vi "rad_FTP Get File Wrapper.vi"(4 "active (F)":bool, 5 "password":string, 6 "binary (T)":bool=TRUE, 8 "error in (no error)":errorcluster, 9 "local path":path=path "C:/Users/bsnover/Desktop/lvappimage.info", 10 "remote path":string="c:\\lvappimage.info", 11 "Target settings":T1={"Hostname"="", "Serial number"="", "Product name"="", "Product code"=0, "System status"="", "Credential type"=enum."None/Unlocked", "User added?"=FALSE, "Primary NIC"={"MAC address"="", "IP Address Request Mode"=2, "IP address"="", "Subnet mask"="", "Gateway"="", "DNS server"=""}} {"Primary NIC"."IP Address Request Mode" items=["Static"=1, "DHCP/Link-Local"=2, "Link-Local Only"=4, "DHCP Only"=8]}) -> (0 "error out":errorcluster)   [LabVIEW 2020]
uses:
  <vilib>/nisyscfg/nisyscfg.lvlib
  <vilib>/nisyscfg/Close (System).vi
  <vilib>/FTP/NI_FTP.lvlib
  Targets/TypeDefs/rad_Target Information.ctl
  Targets/TypeDefs/rad_Target Network Settings.ctl
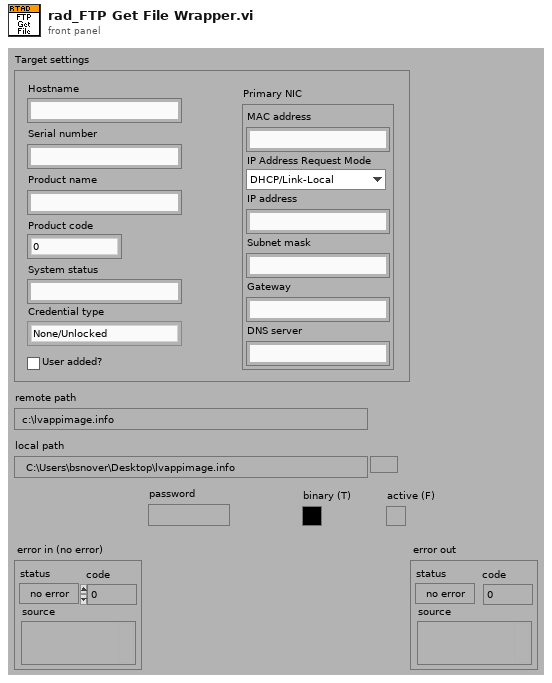
[diagram p1: front panel]
types:
  T1 = typedef "rad_Target Information.ctl" = cluster{"Hostname":string, "Serial number":string, "Product name":string, "Product code":i32, "System status":string, "Credential type":enum16{"None/Unlocked", "FTP Password", "NIAuth Credentials"}, "User added?":bool, "Primary NIC":T2}
  T2 = typedef "rad_Target Network Settings.ctl" = cluster{"MAC address":string, "IP Address Request Mode":i32, "IP address":string, "Subnet mask":string, "Gateway":string, "DNS server":string}
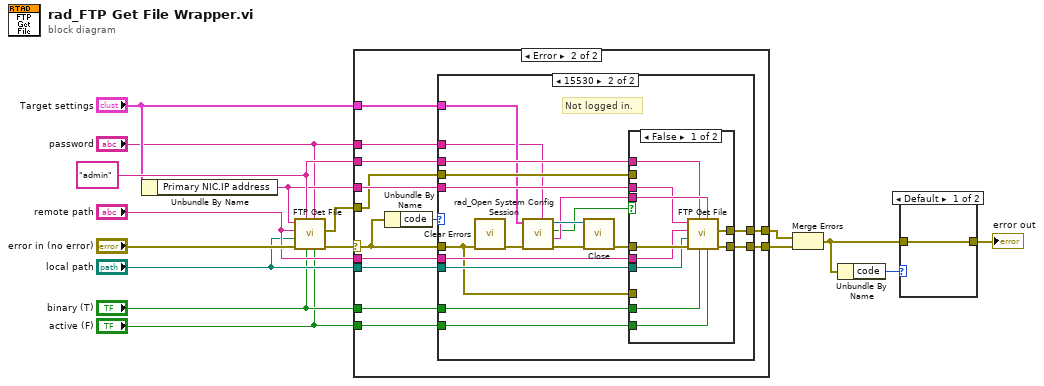
[diagram p0: block diagram]
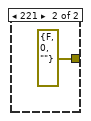
[diagram p5: hidden frame]
diagram:
  w4 = "admin" ("user (admin)")
  n1 = Unbundle By Name("Target settings") -> ("Primary NIC.IP address"=w3:string)
  n2 = call <vilib>:"FTP Get File.vi"("active (T)"="active (F)", "password"="password", "binary (F)"="binary (T)", "user"=w4, "error in (no error)"="error in (no error)", "local path"="local path", "remote path"="remote path", "host"=w3) -> ("error out"=w12:errorcluster, "file error"=w6:errorcluster)  [unwired: 2 in]
  n3 = case shown="Error" w12 {
    selector: w12 -> [w18 w25]
    tunnel: [w18 w31] -> w11
    tunnel: w3 -> [_ w30]
    tunnel: "remote path" -> [_ w29]
    tunnel: "local path" -> [_ w28]
    tunnel: "binary (T)" -> [_ w27]
    tunnel: "active (F)" -> [_ w26]
    tunnel: w6 -> [w17 w23]
    tunnel: [w17 w22] -> w5
    tunnel: w4 -> [_ w21]
    tunnel: "Target settings" -> [_ w20]
    tunnel: "password" -> [_ w19]
    frame No Error {
    }
    frame Error {
      n4 = Unbundle By Name(w25) -> ("code"=w24:i32)
      n5 = case shown="15530" w24 {
        tunnel: w25 -> [w33 w39]
        tunnel: [w33 w47] -> w31
        tunnel: w30 -> [_ w45]
        tunnel: w29 -> [_ w44]
        tunnel: w28 -> [_ w43]
        tunnel: w27 -> [_ w42]
        tunnel: w26 -> [_ w41]
        tunnel: w23 -> [w32 w38]
        tunnel: [w32 w37] -> w22
        tunnel: w21 -> [_ w36]
        tunnel: w20 -> [_ w35]
        tunnel: w19 -> [_ w34]
        frame Default {
        }
        frame 15530 {
          # "Not logged in."
          n6 = call <vilib>:"Clear Errors.vi"("error in (no error)"=w39) -> ("error out"=w49:errorcluster)  [unwired: 5 in, 1 out]
          n7 = call "rad_Open System Config Session.vi"("Password"=w34, "error in (no error)"=w49, "Target settings"=w35) -> ("error out"=w50:errorcluster, "Password out"=w46:string, "Cancelled"=w40:bool, "Session out"=w51:refnum<k21>)  [unwired: 5 in]
          n8 = call-poly <vilib>:"Close.vi"("error in (no error)"=w50, "Session in"=w51) -> ("error out"=w48:errorcluster)  [unwired: 9 in]
          n9 = case shown="False" w40 {
            tunnel: w48 -> [w61 _]
            tunnel: [w60 w63] -> w47
            tunnel: w46 -> [w59 _]
            tunnel: w45 -> [w58 _]
            tunnel: w44 -> [w57 _]
            tunnel: w43 -> [w56 _]
            tunnel: w42 -> [w55 _]
            tunnel: w41 -> [w54 _]
            tunnel: w39 -> [_ w63]
            tunnel: w38 -> [_ w62]
            tunnel: [w53 w62] -> w37
            tunnel: w36 -> [w52 _]
            frame False {
              n10 = call <vilib>:"FTP Get File.vi"("active (T)"=w54, "password"=w59, "binary (F)"=w55, "user"=w52, "error in (no error)"=w61, "local path"=w56, "remote path"=w57, "host"=w58) -> ("error out"=w60:errorcluster, "file error"=w53:errorcluster)  [unwired: 2 in]
            }
            frame True {
            }
          }
        }
      }
    }
  }
  n11 = Merge Errors(w5, w11) -> (w14:errorcluster)
  n12 = Unbundle By Name(w14) -> ("code"=w15:i32)
  n13 = case shown="Default" w15 {
    tunnel: w14 -> [w64 _]
    tunnel: [w64 errorcluster {"status"=FALSE, "code"=0, "source"=""} ("error IO")] -> w13
    frame Default {
    }
    frame 221 {
    }
  }
  "error out" <- w13
